vi "Get Objects in Range.vi"(8 "error in":errorcluster, 9 "End":u16 format="%04x", 10 "Start":u16 format="%04x", 11 "Obj Dict in":refnum<class "Object Dictionary.lvclass">) -> (0 "error out":errorcluster, 2 "Objects in Range":refnum<class "Object Entry.lvclass">[](array[class]), 3 "Obj Dict out":refnum<class "Object Dictionary.lvclass">)   [LabVIEW 2020, in "CANopen.lvlib" / "Object Dictionary.lvclass"]
uses:
  Object Dictionary.lvclass
  Object Dictionary.lvclass/Object Dictionary.ctl
  Ordered-Dictionary/Ordered Object Dictionary/Source/Ordered Object Dictionary.lvclass
  Object Entry/Object Entry.lvclass
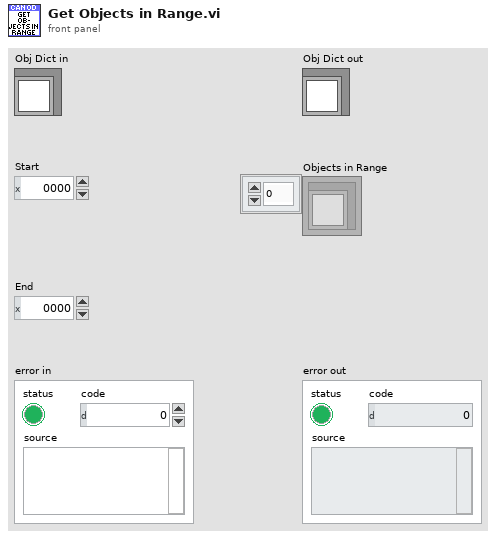
[diagram p1: front panel]
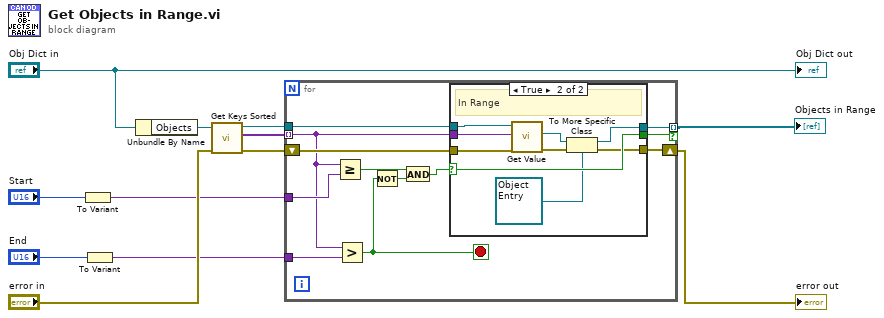
[diagram p0: block diagram]
diagram:
  n1 = To Variant(anything="Start") -> (Variant=w7:variant)
  n2 = To Variant(anything="End") -> (Variant=w5:variant)
  n3 = Unbundle By Name("Obj Dict in") -> ("Objects"=w11:refnum<class "Ordered Object Dictionary.lvclass">)
  n4 = call "Get Keys Sorted.vi"("error in"="error in", "Ordered Object Dictionary in"=w11) -> ("error out"=w3:errorcluster, "Keys Sorted"=w8:variant[], "Ordered Object Dictionary out"=w4:refnum<class "Ordered Object Dictionary.lvclass">)  [unwired: 7 in]
  n5 = for {
    tunnel: w8 -> [w16] mode=indexing
    tunnel: w7 -> [w24]
    tunnel: w5 -> [w23]
    tunnel: w4 -> [w21]
    shift-right: [w19] -> w1
    shift-left: w3 -> [w20]
    tunnel: [w18] -> w2 mode=indexing if=w17
    stop <- w13 stop-if-true
    n6 = Greater Or Equal?(x=w16, y=w24) -> (x >= y?=w22:bool)
    n7 = Greater?(x=w16, y=w23) -> (0:w13:bool)
    n8 = Not(x=w13) -> (.not. x?=w14:bool)
    n9 = And(x=w22, y=w14) -> (x .and. y?=w15:bool)
    n10 = case shown="True" w15 {
      selector: w15 -> [_ w30]
      tunnel: w21 -> [_ w34]
      tunnel: w20 -> [w25 w33]
      tunnel: [w25 w29] -> w19
      tunnel: w16 -> [_ w31]
      tunnel: [_ w30] -> w17
      tunnel: [_ w26] -> w18
      frame False {
      }
      frame True {
        # "In Range"
        n11 = call "Get Value.vi"("error in"=w33, "Key"=w31, "Ordered Object Dictionary in"=w34) -> ("error out"=w32:errorcluster, "Value"=w27:refnum<class>)  [unwired: 6 in, 1 out]
        n12 = To More Specific Class(target class=refnum<class "Object Entry.lvclass"> refnum ("CANopen.lvlib:Obj Entry"), reference=w27, error in=w32) -> (specific class reference=w26:refnum<class "Object Entry.lvclass">, error out=w29:errorcluster)
      }
    }
  }
  "error out" <- w1
  "Objects in Range" <- w2
  "Obj Dict out" <- "Obj Dict in"
